vi "Send Data.vi"(8 "error in":errorcluster, 10 "Data":string, 11 "connection ID In":refnum<k5>) -> (0 "error out":errorcluster, 3 "connection ID Out":refnum<k5>)   [LabVIEW 2018, in "Labview Python.lvlib"]
uses:
  Labview Python.lvlib
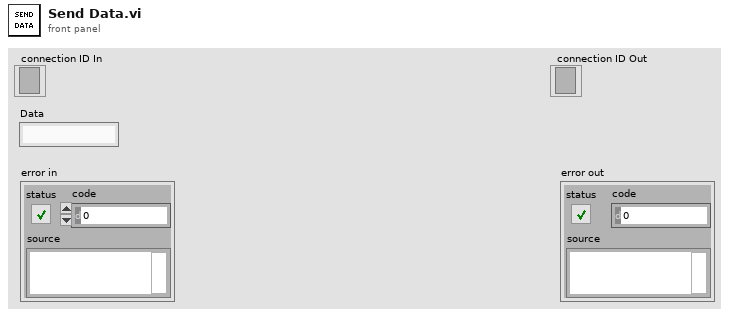
[diagram p1: front panel]
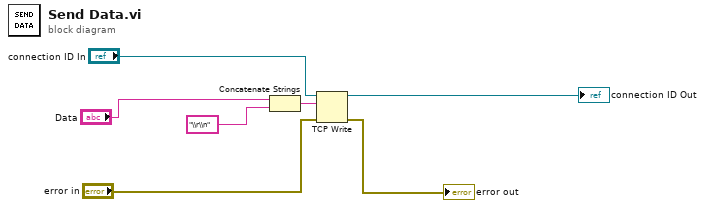
[diagram p0: block diagram]
diagram:
  n1 = Concatenate Strings("Data", "\\r\\n") -> (w7:string)
  n2 = TCP Write(connection ID="connection ID In", data in=w7, error in (no error)="error in") -> (connection ID out=→"connection ID Out":refnum<k5>, error out=→"error out":errorcluster)  [unwired: 2 out]
